vi "LoadFromINI.vi"(8 "error in (no error)":errorcluster, 10 "Path Control":path, 11 "reference in":refnum<class "Timing.lvclass">) -> (0 "error out":errorcluster, 3 "reference out":refnum<class "Timing.lvclass">)   [LabVIEW 2019, in "Timing.lvclass"]
uses:
  Timing.lvclass
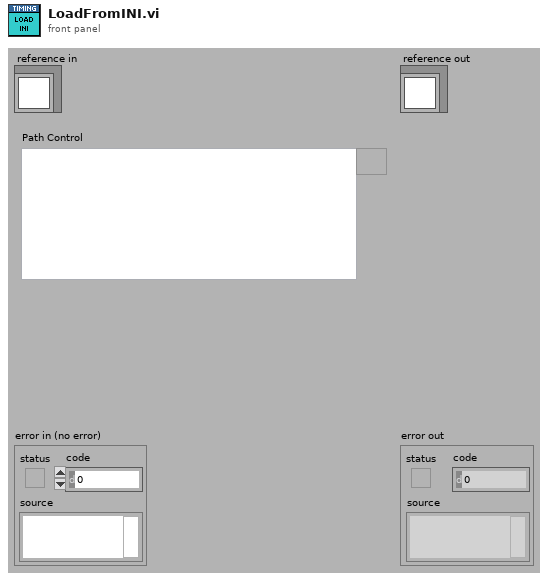
[diagram p1: front panel]
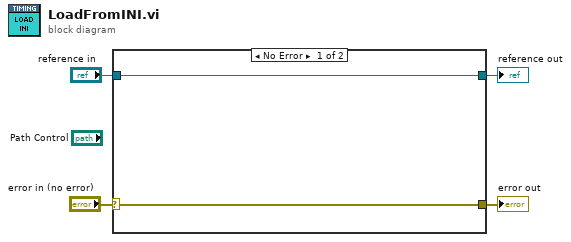
[diagram p0: block diagram]
diagram:
  n1 = case shown="No Error" "error in (no error)" {
    selector: "error in (no error)" -> [w5 w8]
    tunnel: [w5 w8] -> w3
    tunnel: [w6 w7] -> w1
    tunnel: "reference in" -> [w6 w7]
    frame No Error {
    }
    frame Error {
    }
  }
  "error out" <- w3
  "reference out" <- w1
